vi "basic query test.vi"() -> ()   [LabVIEW 2020, in "mysql.lvlib" / "mysql.lvclass"]
uses:
  mysql.net/mysql.lvclass
  5b913561-ff12-4fa5-a3bd-0912ab83ba32.vi
  <vilib>/Utility/error.llb/Error Cluster From Error Code.vi
panel:
  out "Result":string[][](array[string])=[["1", "3.99"], ["2", "10.99"], ["3", "1.69"], ["4", "19.95"]]
  in  "Connection string":string="server=127.0.0.1;uid=root;pwd=Nitrog3n;database=test"
  in  "error in (no error)":errorcluster
  out "error out":errorcluster
  in  "Query string":string="SELECT article, MAX(price) AS price\nFROM   shop\nGROUP BY article;"
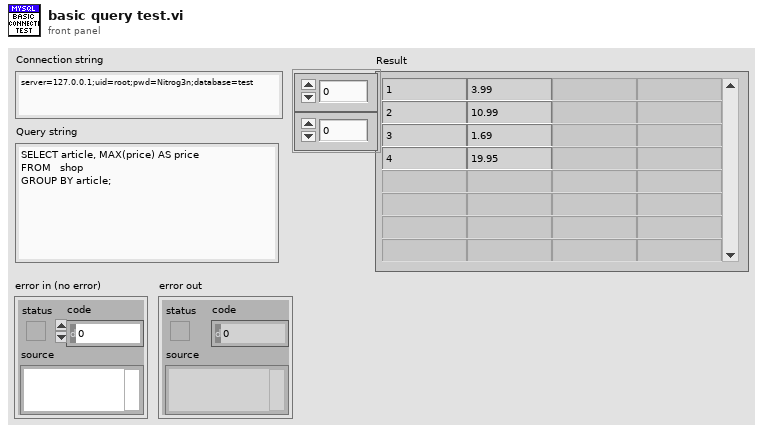
[diagram p1: front panel]
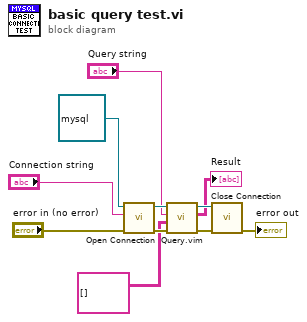
[diagram p0: block diagram]
diagram:
  n1 = call-dynamic "Open Connection.vi"("error in (no error)"="error in (no error)", "Connection string"="Connection string", "mysql in"=refnum<class "mysql.lvclass"> refnum) -> ("error out"=w10:errorcluster, "mysql out"=w11:refnum<class "mysql.lvclass">)  [unwired: 7 in]
  n2 = call "Query.vim"("error in (no error)"=w10, "Type and Default"=string[][] [] ("Result 2"), "Query string"="Query string", "IDatabase in"=w11) -> ("error out"=w8:errorcluster, "Result"=→"Result":string[][], "IDatabase out"=w9:refnum<class "mysql.lvclass">)  [unwired: 5 in]
  n3 = call-dynamic "Close Connection.vi"("error in (no error)"=w8, "mysql in"=w9) -> ("error out"=→"error out":errorcluster)  [unwired: 8 in, 1 out]
